vi "ParseDataSetRequest.vi"(8 "error in (no error)":errorcluster, 9 "message":T1, 10 "config":T4, 11 "Qbus in":refnum<class "Qbus.lvclass">) -> (0 "error out":errorcluster, 2 "config out":T4)   [LabVIEW 2017, in "EmsaTestPanel.lvlib"]
uses:
  <vilib>/addons/InsightCM/Devices/Shared/Emsa/EmsaTestPanel/EmsaTestPanel.lvlib
  <vilib>/addons/Qbus/Qbus.lvclass
  <vilib>/addons/InsightCM/Devices/Shared/Emsa/EmsaTestPanel/controls/Configuration.ctl
  <vilib>/addons/InsightCM/Devices/Shared/Emsa/EmsaTestPanel/controls/DataSetType.ctl
  <vilib>/addons/InsightCM/Devices/Shared/Common/TestPanel/controls/Configuration.ctl
  <vilib>/addons/InsightCM/Devices/Shared/Common/TestPanel/controls/State.ctl
  <vilib>/addons/InsightCM/MessageBus/Base/controls/IRoutingSource.ctl
  <vilib>/addons/InsightCM/MessageBus/Base/controls/Message.ctl
  <vilib>/addons/InsightCM/MessageBus/Base/controls/MessageHeader.ctl
  <vilib>/addons/InsightCM/MessageBus/Base/controls/KeyValuePair.ctl
  <vilib>/addons/InsightCM/Devices/Shared/Emsa/EmsaAcquisition/controls/StartOnDemandAcquisitionRoutedMessage.ctl
  <vilib>/addons/InsightCM/Devices/Shared/Common/TestPanel/TestPanel.lvlib
  <vilib>/addons/InsightCM/Utilities/PropertyHelpers/PropertyHelpers.lvlib
  <vilib>/addons/InsightCM/Devices/Shared/Emsa/EmsaAcquisition/EmsaAcquisition.lvlib
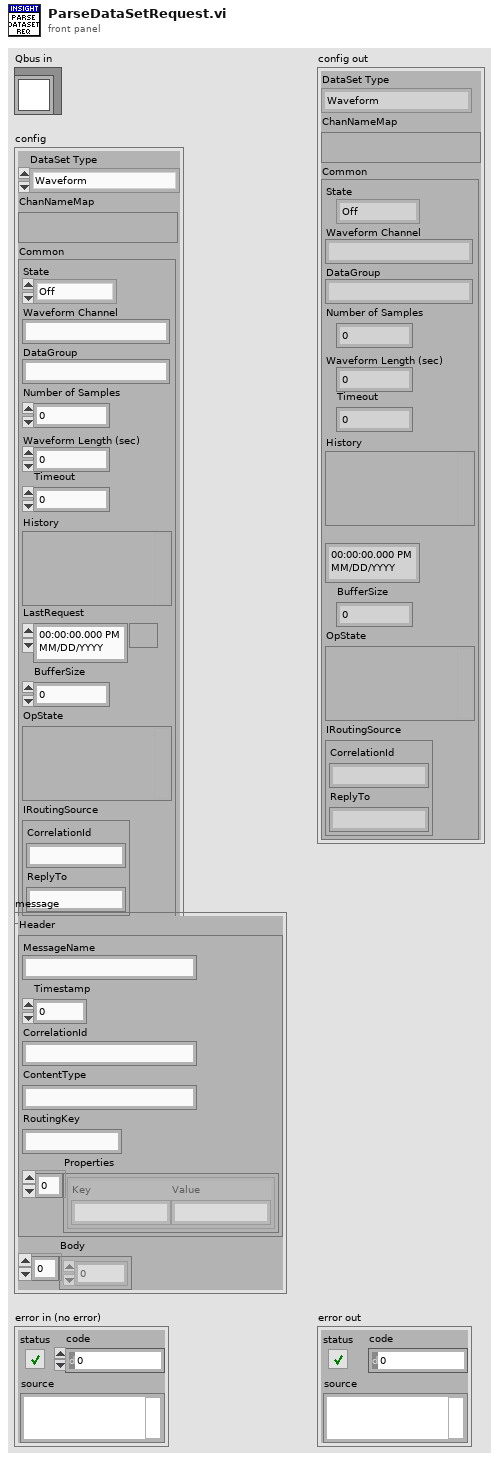
[diagram p1: front panel]
types:
  T1 = typedef "Message.ctl" = cluster{"Header":T2, "Body":u8[]}
  T2 = typedef "MessageHeader.ctl" = cluster{"MessageName":string, "Timestamp":i64, "CorrelationId":string, "ContentType":string, "RoutingKey":string, "Properties":T3[]}
  T3 = typedef "KeyValuePair.ctl" = cluster{"Key":string, "Value":string}
  T4 = typedef "EmsaTestPanel.lvlib/Configuration.ctl" = cluster{"DataSet Type":T5, "ChanNameMap":variant, "Common":T6}
  T5 = typedef "EmsaTestPanel.lvlib/DataSetType.ctl" = enum16{"Waveform", "Sweep", "WAV"}
  T6 = typedef "TestPanel.lvlib/Configuration.ctl" = cluster{"State":T7, "Waveform Channel":string, "DataGroup":string, "Number of Samples":i32, "Waveform Length (sec)":dbl, "Timeout":dbl, "History":variant, "LastRequest":timestamp, "BufferSize":i32, "OpState":variant, "IRoutingSource":T8}
  T7 = typedef "TestPanel.lvlib/State.ctl" = enum16{"Off", "On", "PendingValues", "PendingDataSet"}
  T8 = typedef "IRoutingSource.ctl" = cluster{"CorrelationId":string, "ReplyTo":string}
  T9 = typedef "DeviceTestPanelGetDataSetForChannelRequestBody.ctl" = cluster{"DataGroup":string, "ChannelName":string, "Properties":T3[]}
  T10 = typedef "EmsaAcquisition.lvlib/StartOnDemandAcquisitionRoutedMessage.ctl" = cluster{"Channel Name":string, "Audio":bool, "Center Frequency":dbl, "Bandwidth":dbl, "Duration":dbl, "Reference Level":dbl}
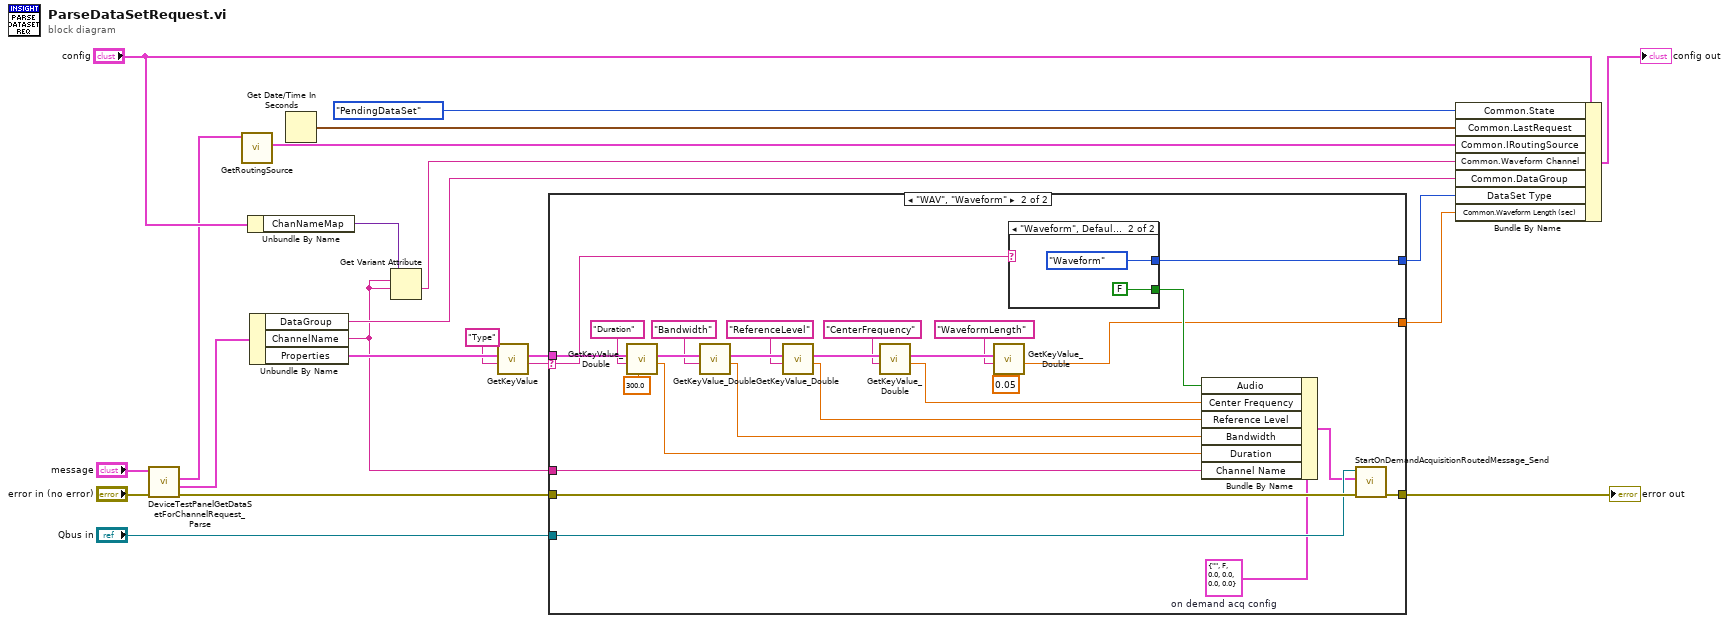
[diagram p0: block diagram]
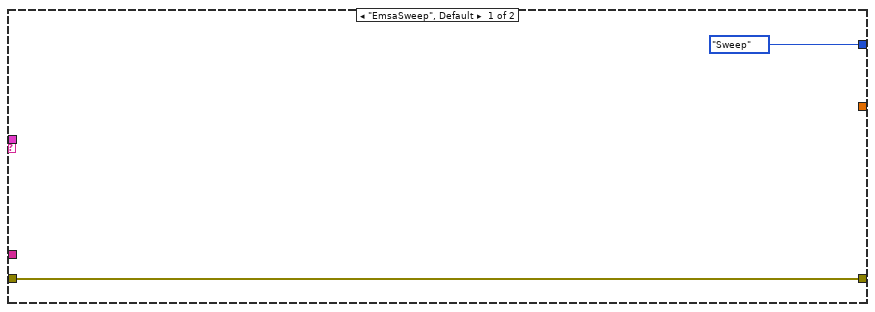
[diagram p2: hidden frame]
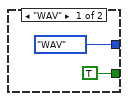
[diagram p3: hidden frame]
diagram:
  n1 = call <vilib>:"DeviceTestPanelGetDataSetForChannelRequest_Parse.vi"("error in (no error)"="error in (no error)", "Message"="message") -> ("error out"=w5:errorcluster, "Body"=w15:T9, "Header"=w18:T2)  [unwired: 6 in, 1 out]
  n2 = call <vilib>:"GetRoutingSource.vi"("Header in"=w18) -> ("IRoutingSource"=w19:T8)  [unwired: 9 in, 1 out]
  n3 = Unbundle By Name("config") -> ("ChanNameMap"=w21:variant)
  n4 = Unbundle By Name(w15) -> ("DataGroup"=w12:string, "ChannelName"=w3:string, "Properties"=w11:T3[])
  n5 = Get Date/Time In Seconds() -> (seconds since 1Jan1904=w17:timestamp)
  n6 = Get Variant Attribute(Variant=w21, name=w3, default value (empty Variant)=w3) -> (value=w22:string)  [unwired: 1 in, 3 out]
  n7 = call <vilib>:"GetKeyValue.vi"("key"="Type", "key value pairs"=w11) -> ("value"=w9:string, "key value pairs out"=w8:T3[])  [unwired: 7 in, 1 out]
  n8 = case shown="\"WAV\", \"Waveform\"" w9 {
    selector: w9 -> [_ w48]
    tunnel: w8 -> [_ w49]
    tunnel: [DataSetType."Sweep" ("DataSet Type") w50] -> w7
    tunnel: [w23 w40] -> w6
    tunnel: w5 -> [w23 w39]
    tunnel: "Qbus in" -> [_ w38]
    tunnel: w3 -> [_ w36]
    tunnel: [_ w26] -> w1
    frame "EmsaSweep", Default {
    }
    frame "WAV", "Waveform" {
      w37 = T10 {"Channel Name"="", "Audio"=FALSE, "Center Frequency"=0.0, "Bandwidth"=0.0, "Duration"=0.0, "Reference Level"=0.0}  # on demand acq config
      n9 = call <vilib>:"GetKeyValue_Double.vi"("default"=300.0, "key"="Duration", "key value pairs"=w49) -> ("value"=w35:dbl, "key value pairs out"=w47:T3[])  [unwired: 6 in, 1 out]
      n10 = call <vilib>:"GetKeyValue_Double.vi"("key"="Bandwidth", "key value pairs"=w47) -> ("value"=w33:dbl, "key value pairs out"=w46:T3[])  [unwired: 7 in, 1 out]
      n11 = call <vilib>:"GetKeyValue_Double.vi"("key"="ReferenceLevel", "key value pairs"=w46) -> ("value"=w32:dbl, "key value pairs out"=w45:T3[])  [unwired: 7 in, 1 out]
      n12 = call <vilib>:"GetKeyValue_Double.vi"("key"="CenterFrequency", "key value pairs"=w45) -> ("value"=w31:dbl, "key value pairs out"=w28:T3[])  [unwired: 7 in, 1 out]
      n13 = call <vilib>:"GetKeyValue_Double.vi"("default"=0.05, "key"="WaveformLength", "key value pairs"=w28) -> ("value"=w26:dbl)  [unwired: 6 in, 2 out]
      n14 = case shown="\"Waveform\", Default" w48 {
        tunnel: [DataSetType."WAV" ("DataSet Type") DataSetType."Waveform" ("DataSet Type")] -> w50
        tunnel: [TRUE ("Audio") FALSE ("Audio")] -> w30
        frame "WAV" {
        }
        frame "Waveform", Default {
        }
      }
      n15 = Bundle By Name(cluster=w37, "Audio"=w30, "Center Frequency"=w31, "Reference Level"=w32, "Bandwidth"=w33, "Duration"=w35, "Channel Name"=w36) -> (w29:T10)
      n16 = call <vilib>:"StartOnDemandAcquisitionRoutedMessage_Send.vi"("error in (no error)"=w39, "on demand acq config"=w29, "Qbus in"=w38) -> ("error out"=w40:errorcluster)  [unwired: 7 in, 1 out]
    }
  }
  "error out" <- w6
  n17 = Bundle By Name(cluster="config", "Common.State"=State."PendingDataSet" ("Test Panel State"), "Common.LastRequest"=w17, "Common.IRoutingSource"=w19, "Common.Waveform Channel"=w22, "Common.DataGroup"=w12, "DataSet Type"=w7, "Common.Waveform Length (sec)"=w1) -> (→"config out":T4)
